vi "therm sim globals.vi"() -> ()   [LabVIEW 2016]
panel:
  in  "insulation":enum16{"uncovered", "covered"}(ring)=enum."covered"
  in  "air speed":dbl
  in  "Power":dbl=0.3259911894273128 format="%#_4g"
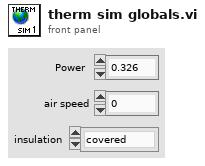
[diagram p1: front panel]
diagram:
